vi "FTW-Message-Lossy-Construct.vi"(9 "max queue size (1)":i32=1, 11 "error in":errorcluster) -> (4 "FTW-Message-Lossy":refnum<class "FTW-Message-Lossy.lvclass">, 15 "error out":errorcluster)   [LabVIEW 2015, in "FTW-Message-Lossy.lvclass"]
uses:
  FTW-Message-Lossy.lvclass
  FTW-Message-Lossy.lvclass/FTW-Message-Lossy.ctl
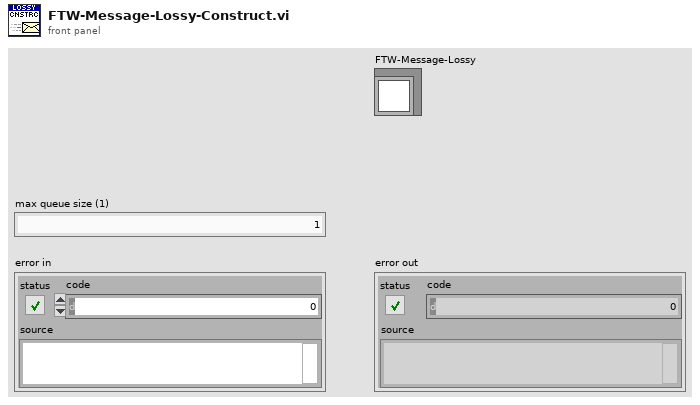
[diagram p1: front panel]
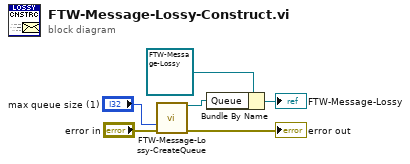
[diagram p0: block diagram]
diagram:
  n1 = call "FTW-Message-Lossy-CreateQueue.vi"("max queue size (1)"="max queue size (1)", "error in"="error in") -> ("Queue"=w4:refnum<queue>, "error out"=→"error out":errorcluster)  [unwired: 12 in]
  n2 = Bundle By Name(cluster=refnum<class "FTW-Message-Lossy.lvclass"> refnum ("FTW-Message-Lossy"), "Queue"=w4) -> (→"FTW-Message-Lossy":refnum<class "FTW-Message-Lossy.lvclass">)
